vi "DTtoASCII.vi"(3 "Slide":dbl(slide) scale=0.0..100.0) -> (0 "Numeric":dbl, 1 "ASCII":string)   [LabVIEW 2014]
panel:
  in  "Channel":dbl=1.0 min=1.0 max=2.0 step=1.0
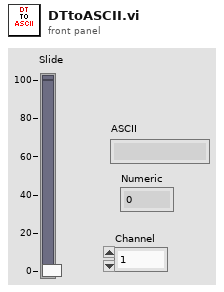
[diagram p1: front panel]
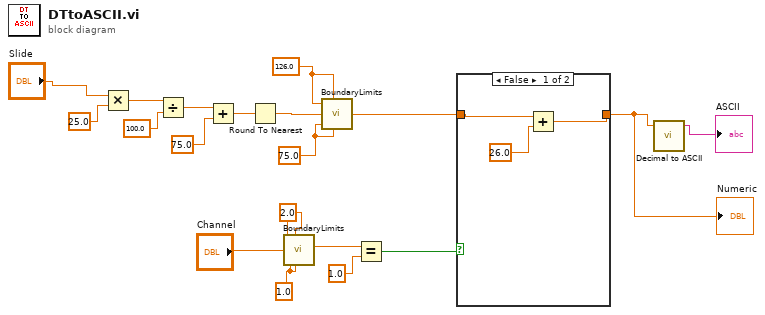
[diagram p0: block diagram]
diagram:
  w10 = 2.0
  w8 = 1.0
  w16 = 126.0
  w14 = 75.0
  n1 = Multiply(x="Slide", y=25.0) -> (x*y=w19:dbl)
  n2 = Divide(x=w19, y=100.0) -> (x/y=w18:dbl)
  n3 = Add(x=w18, y=75.0) -> (x+y=w17:dbl)
  n4 = Round To Nearest(number=w17) -> (nearest integer value=w15:dbl)
  n5 = call "BoundaryLimits.vi"("UpperLimit"=w10, "UpperValue"=w10, "Input"="Channel", "LowerLimit"=w8, "LowerValue"=w8) -> ("Output"=w6:dbl)
  n6 = call "BoundaryLimits.vi"("UpperLimit"=w16, "UpperValue"=w16, "Input"=w15, "LowerLimit"=w14, "LowerValue"=w14) -> ("Output"=w3:dbl)
  n7 = Equal?(x=w6, y=1.0) -> (x = y?=w4:bool)
  n8 = case shown="False" w4 {
    tunnel: [w20 w23] -> w1
    tunnel: w3 -> [w21 w23]
    frame False {
      n9 = Add(x=w21, y=26.0) -> (x+y=w20:dbl)
    }
    frame True {
    }
  }
  "Numeric" <- w1
  n10 = call "Decimal to ASCII.vi"("Decimal Number"=w1) -> ("Decimal String"=→"ASCII":string)  [unwired: 2 in, 2 out]
